vi "Message Handler.vi"(7 "Action":T5, 8 "Error In":errorcluster, 9 "Writing Timeout (0)":i32, 11 "Message":T1) -> (0 "Error Out":errorcluster, 1 "# elements remaining":i32, 3 "Message Out":T1)   [LabVIEW 2024, in "Road.lvlib" / "GUI.lvlib"]
doc: "------------------------------------\nLast Modified <B>2025 March 30th</B> by: maj@agh.edu.pl"
uses:
  GUI.lvlib
  #typedef_CommunicationModuleAction.ctl
  #typedef_Message.ctl
  #typedef_MessageCommand.ctl
  #typedef_MessageParameters.ctl
  #typedef_MessageEnum.ctl
panel:
  # "Inputs"
  # "Outputs"
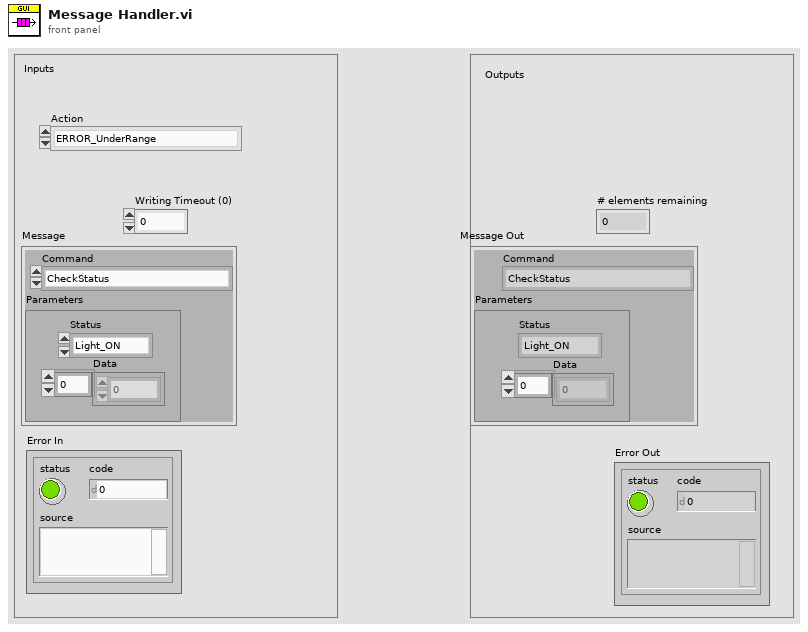
[diagram p1: front panel]
types:
  T1 = typedef "Road.lvlib/GUI.lvlib/#typedef_Message.ctl" = cluster{"Command":T2, "Parameters":T3}
  T2 = typedef "Road.lvlib/GUI.lvlib/#typedef_MessageCommand.ctl" = enum16{"CheckStatus", "NewData", "ShutDown"}
  T3 = typedef "Road.lvlib/GUI.lvlib/#typedef_MessageParameters.ctl" = cluster{"Status":T4, "Data":dbl[]}
  T4 = typedef "#typedef_MessageEnum.ctl" = enum16{"Light_ON", "IDLE", "Brakdown_ON", "Breakdown_OFF"}
  T5 = typedef "Road.lvlib/GUI.lvlib/#typedef_CommunicationModuleAction.ctl" = enum16{"ERROR_UnderRange", "Init", "Connect To existing", "Send Msg", "Priority Send", "Receive Msg", "Preview Messages", "ErrorHandle", "ShutDown", "ERROR_OverRange"}
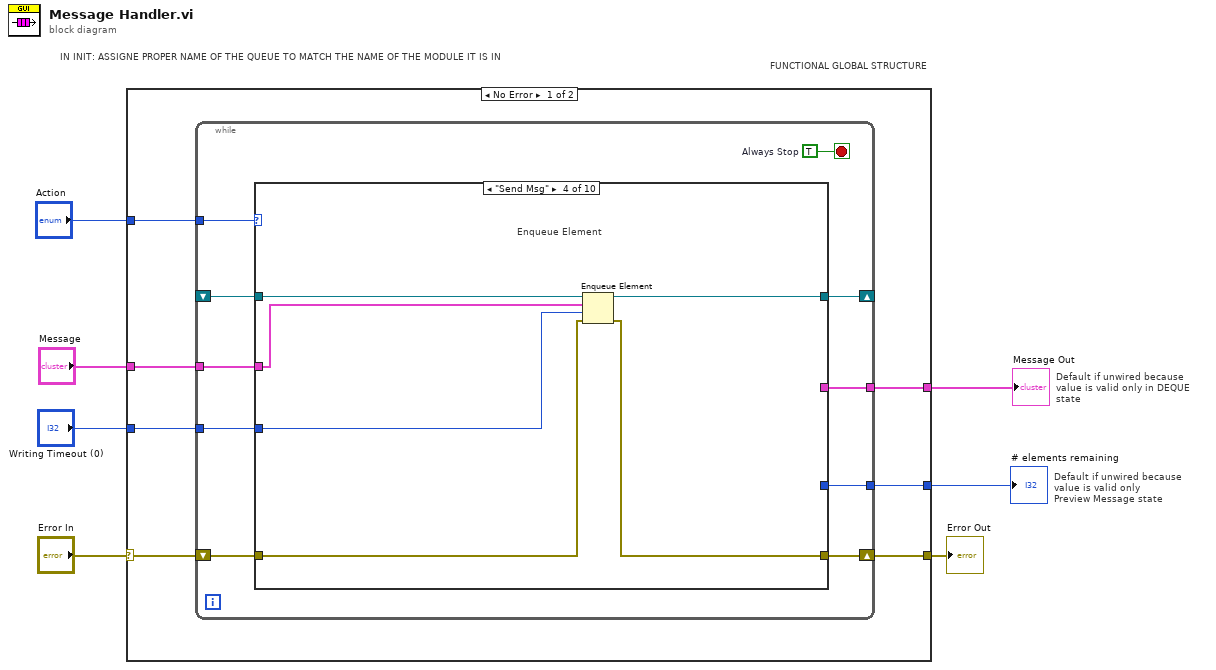
[diagram p0: block diagram]
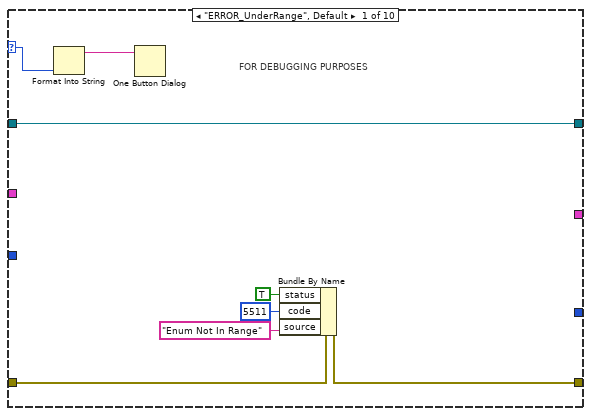
[diagram p2: hidden frame]
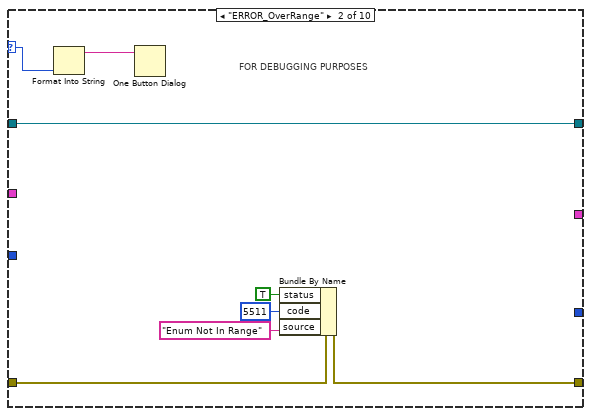
[diagram p3: hidden frame]
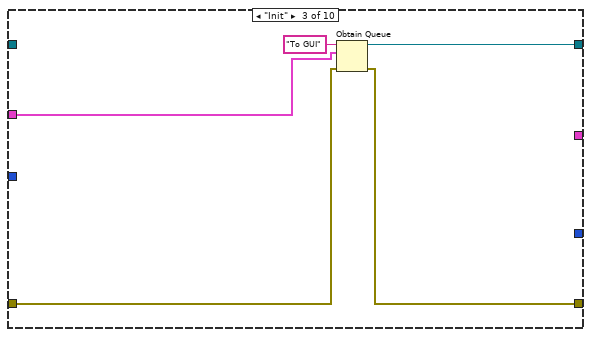
[diagram p4: hidden frame]
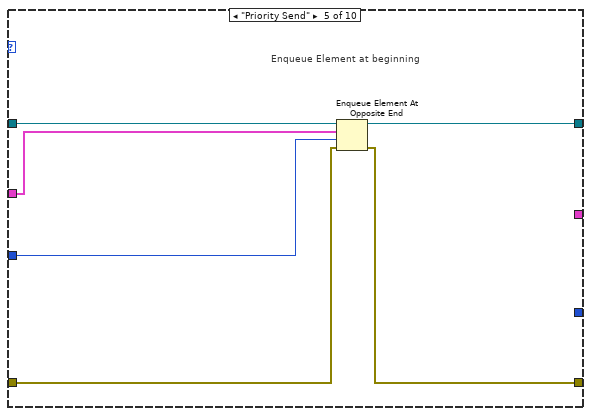
[diagram p5: hidden frame]
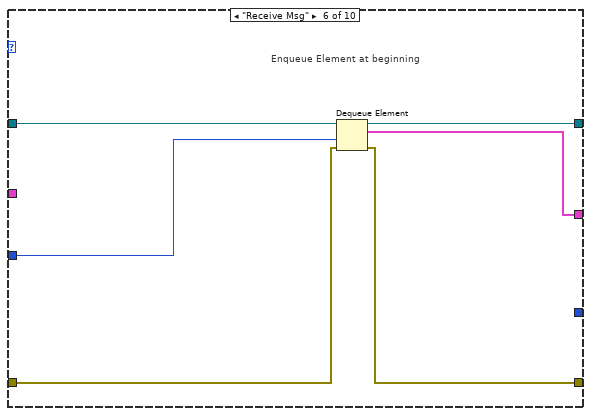
[diagram p6: hidden frame]
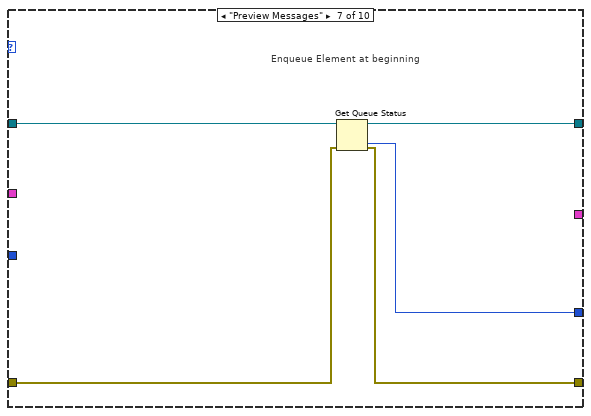
[diagram p7: hidden frame]
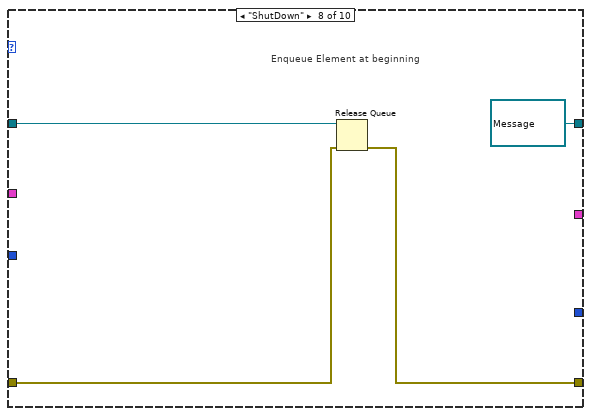
[diagram p8: hidden frame]
diagram:
  # "IN INIT: ASSIGNE PROPER NAME OF THE QUEUE TO MATCH THE NAME OF THE MODULE IT IS IN"
  # "Default if unwired because value is valid only \nPreview Message state"
  # "Default if unwired because value is valid only in DEQUE state"
  # "FUNCTIONAL GLOBAL STRUCTURE"
  n1 = case shown="No Error" "Error In" {
    selector: "Error In" -> [w13 w77]
    tunnel: [w14 w77] -> w6
    tunnel: "Action" -> [w12 _]
    tunnel: "Message" -> [w11 _]
    tunnel: "Writing Timeout (0)" -> [w10 _]
    tunnel: [w9 _] -> w2
    tunnel: [w8 _] -> w1
    frame No Error {
      n2 = while {
        shift-right: [w23] -> w14
        shift-left: w13 -> [w22]
        tunnel: w12 -> [w21]
        shift-right: [w20] -> _
        shift-left: _ -> [w19]
        tunnel: w11 -> [w18]
        tunnel: w10 -> [w17]
        tunnel: [w16] -> w9
        tunnel: [w15] -> w8
        stop <- w24 stop-if-true
        w24 = TRUE  # Always Stop
        n3 = case shown="\"Send Msg\"" w21 {
          selector: w21 -> [w30 w38 _ _ _ _ _ _ _ _]
          tunnel: [w28 w36 w43 w50 w56 w63 w68 w69 w73 w75] -> w23
          tunnel: w22 -> [w32 w40 w44 w51 w57 w60 w65 w71 w73 w75]
          tunnel: [w31 w39 w41 w48 w54 w62 w67 refnum<queue> refnum ("Queue IN") w74 w76] -> w20
          tunnel: w19 -> [w31 w39 _ w47 w53 w61 w66 w72 w74 w76]
          tunnel: w18 -> [_ _ w42 w49 w55 _ _ _ _ _]
          tunnel: w17 -> [_ _ _ w46 w52 w59 _ _ _ _]
          tunnel: [_ _ _ _ _ w58 _ _ _ _] -> w16
          tunnel: [_ _ _ _ _ _ w64 _ _ _] -> w15
          frame "ERROR_UnderRange", Default {
            # "FOR DEBUGGING PURPOSES"
            n4 = Format Into String(w30) -> (resulting string=w29:string)  [unwired: 3 in, 1 out]
            n5 = One Button Dialog(message=w29) -> ()  [unwired: 1 in, 1 out]
            n6 = Bundle By Name(cluster=w32, "status"=TRUE, "code"=5511, "source"="Enum Not In Range") -> (w28:errorcluster)
          }
          frame "ERROR_OverRange" {
            # "FOR DEBUGGING PURPOSES"
            n7 = Format Into String(w38) -> (resulting string=w37:string)  [unwired: 3 in, 1 out]
            n8 = One Button Dialog(message=w37) -> ()  [unwired: 1 in, 1 out]
            n9 = Bundle By Name(cluster=w40, "status"=TRUE, "code"=5511, "source"="Enum Not In Range") -> (w36:errorcluster)
          }
          frame "Init" {
            n10 = Obtain Queue(name (unnamed)="To GUI", element data type=w42, error in (no error)=w44) -> (queue out=w41:refnum<queue>, error out=w43:errorcluster)  [unwired: 2 in, 1 out]
          }
          frame "Send Msg" {
            # "Enqueue Element"
            n11 = Enqueue Element(queue=w47, element=w49, timeout in ms (-1)=w46, error in (no error)=w51) -> (queue out=w48:refnum<queue>, error out=w50:errorcluster)  [unwired: 1 out]
          }
          frame "Priority Send" {
            # "Enqueue Element at beginning"
            n12 = Enqueue Element At Opposite End(queue=w53, element=w55, timeout in ms (-1)=w52, error in (no error)=w57) -> (queue out=w54:refnum<queue>, error out=w56:errorcluster)  [unwired: 1 out]
          }
          frame "Receive Msg" {
            # "Enqueue Element at beginning"
            n13 = Dequeue Element(queue=w61, timeout in ms (-1)=w59, error in (no error)=w60) -> (queue out=w62:refnum<queue>, element=w58:T1, error out=w63:errorcluster)  [unwired: 1 out]
          }
          frame "Preview Messages" {
            # "Enqueue Element at beginning"
            n14 = Get Queue Status(queue=w66, error in (no error)=w65) -> (queue out=w67:refnum<queue>, error out=w68:errorcluster, # elements in queue=w64:i32)  [unwired: 1 in, 5 out]
          }
          frame "ShutDown" {
            # "Enqueue Element at beginning"
            n15 = Release Queue(queue=w72, error in (no error)=w71) -> (error out=w69:errorcluster)  [unwired: 1 in, 2 out]
          }
          frame "ErrorHandle" {
            # "Developer: This state is reserved for future usage as ALL modules should handle their own errors"
          }
          frame "Connect To existing" {
            # "If QUEUE Created in different pace the reference can be stored here locally"
          }
        }
      }
    }
    frame Error {
    }
  }
  "Error Out" <- w6
  "Message Out" <- w2
  "# elements remaining" <- w1
